vi "example_vi_2.vi"() -> ()   [LabVIEW 2015]
panel:
  out "max array value":u8
  out "new boolean":bool
  out "new string":string
  out "new number":dbl
  out "array element":u8
  out "new array":u8[](array[slide]) scale=0.0..100.0
  in  "starting string":string
  in  "starting boolean":bool
  in  "starting number":dbl
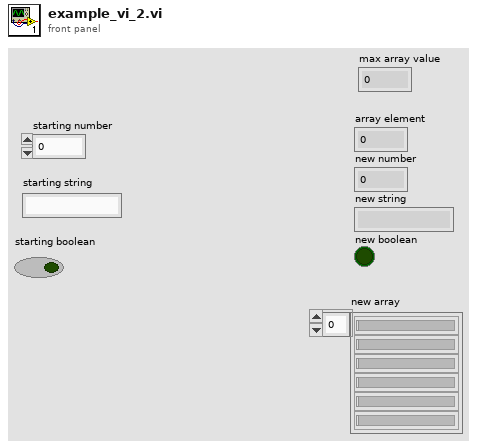
[diagram p1: front panel]
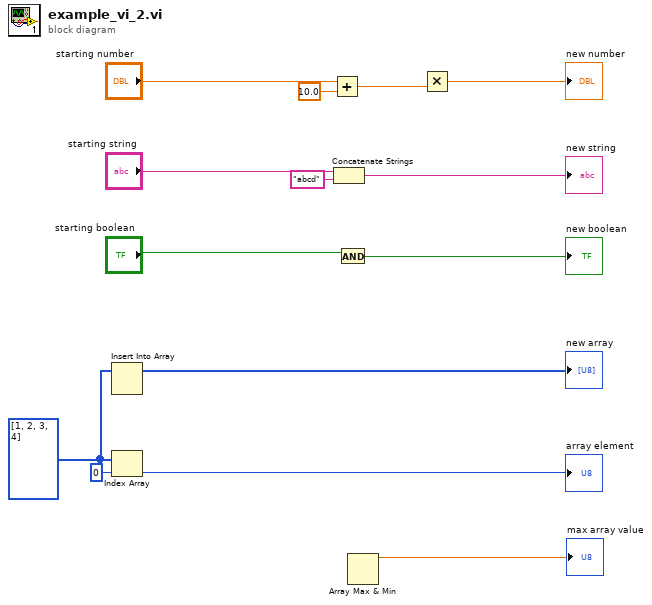
[diagram p0: block diagram]
diagram:
  w11 = u8[] [1, 2, 3, 4]
  n1 = Insert Into Array(array=w11) -> (→"new array":u8[])  [unwired: 2 in]
  n2 = Index Array(array=w11, index=0) -> (element=→"array element":u8)
  n3 = Add(x="starting number", y=10.0) -> (x+y=w3:dbl)
  n4 = Concatenate Strings("starting string", "abcd" ("string")) -> (→"new string":string)
  n5 = And(x="starting boolean") -> (x .and. y?=→"new boolean":bool)  [unwired: 1 in]
  n6 = Array Max & Min() -> (max value=→"max array value":dbl)  [unwired: 1 in, 3 out]
  n7 = Multiply(y=w3) -> (x*y=→"new number":dbl)  [unwired: 1 in]
